vi "EASY-DRIVER Example.vi"() -> ()   [LabVIEW 2020, in "CAENels EASY-DRIVER.lvlib"]
doc: "When the example is executed, it sets the FAST-PS to CV mode and updates the set-point 10 times per second."
uses:
  CAENels EASY-DRIVER.lvlib
panel:
  out "Output Current Chart":dbl(graph)
  out "Fault condition":bool
  out "ON/OFF":bool
  out "Module Status":string="0"
  out "Output Voltage":string="0"
  out "Output Current":string="0"
  in  "Current Setpoint":dbl step=0.1
  in  "Stop Button":bool
  in  "IP address":string="192.168.0.10"
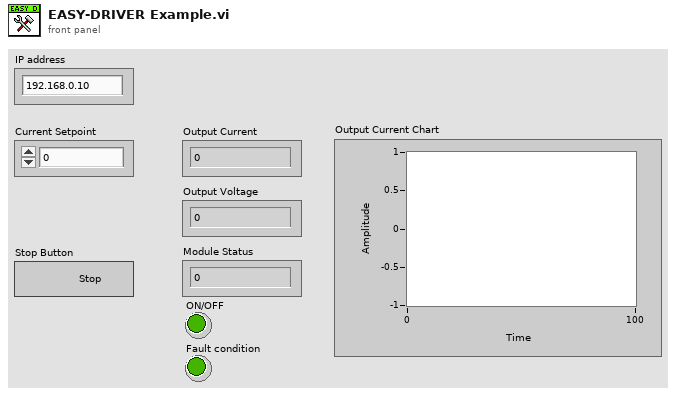
[diagram p1: front panel]
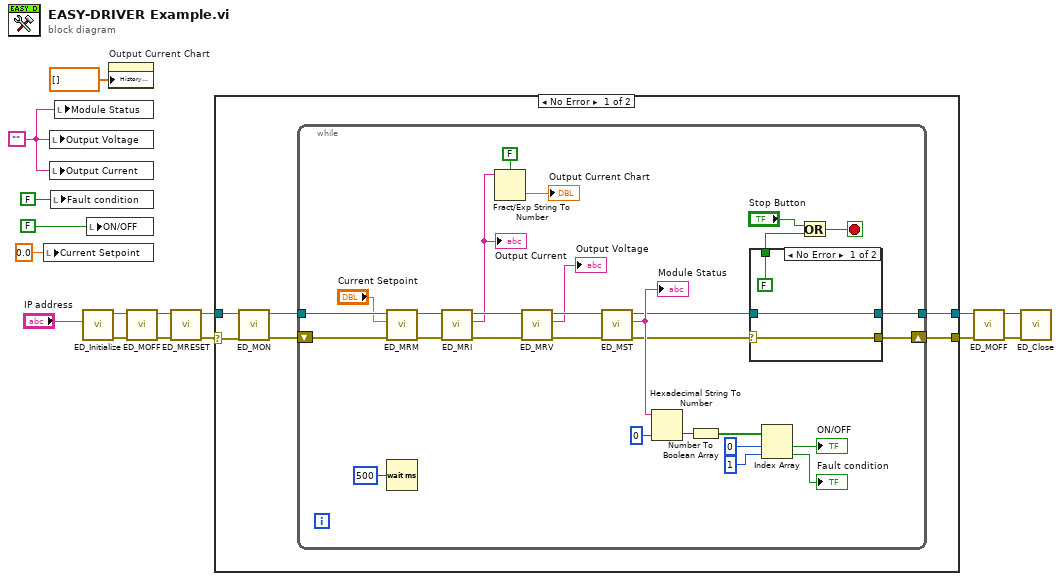
[diagram p0: block diagram]
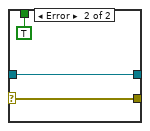
[diagram p2: hidden frame]
diagram:
  w2 = ""
  n1 = local write "Current Setpoint"(0.0 ("Current Setpoint")) -> ()
  n2 = local write "Output Voltage"(w2) -> ()
  n3 = local write "Output Current"(w2) -> ()
  n4 = local write "Fault condition"(FALSE ("Fault condition")) -> ()
  n5 = local write "Module Status"(w2) -> ()
  n6 = call "ED_Initialize.vi"("IP address"="IP address") -> ("error out"=w15:errorcluster, "connection ID"=w14:refnum<k5>)  [unwired: 5 in]
  n7 = local write "ON/OFF"(FALSE ("ON/OFF")) -> ()
  n8 = property on="Output Current Chart" class="WFChart (strict)"("History Data"=dbl[] []) -> ()  [unwired: 2 in, 2 out]
  n9 = call "ED_MOFF.vi"("error in (no error)"=w15, "connection ID"=w14) -> ("error out"=w12:errorcluster, "connection ID out"=w13:refnum<k5>)  [unwired: 4 in]
  n10 = call "ED_MRESET.vi"("error in (no error)"=w12, "connection ID"=w13) -> ("error out"=w3:errorcluster, "connection ID out"=w7:refnum<k5>)  [unwired: 4 in]
  n11 = case shown="No Error" w3 {
    selector: w3 -> [w17 w58]
    tunnel: [w19 w58] -> w9
    tunnel: [w18 w59] -> w8
    tunnel: w7 -> [w22 w59]
    frame No Error {
      n12 = call "ED_MON.vi"("error in (no error)"=w17, "connection ID"=w22) -> ("error out"=w20:errorcluster, "connection ID out"=w21:refnum<k5>)  [unwired: 4 in]
      n13 = while {
        tunnel: w21 -> [w49]
        shift-right: [w31] -> w19
        shift-left: w20 -> [w50]
        tunnel: [w30] -> w18
        stop <- w27 stop-if-true
        n14 = call "ED_MRM.vi"("error in (no error)"=w50, "current"="Current Setpoint", "connection ID"=w49) -> ("error out"=w47:errorcluster, "connection ID out"=w48:refnum<k5>)  [unwired: 3 in]
        n15 = Wait (ms)(milliseconds to wait=u32 500) -> ()  [unwired: 1 out]
        n16 = call "ED_MRI.vi"("error in (no error)"=w47, "connection ID"=w48) -> ("error out"=w45:errorcluster, "current"=w25:string, "connection ID out"=w46:refnum<k5>)  [unwired: 3 in]
        "Output Current" <- w25
        n17 = Fract/Exp String To Number(use system decimal point (T)=FALSE, string=w25) -> (number=→"Output Current Chart":dbl)  [unwired: 2 in, 1 out]
        n18 = call "ED_MRV.vi"("error in (no error)"=w45, "connection ID"=w46) -> ("error out"=w43:errorcluster, "voltage"=→"Output Voltage":string, "connection ID out"=w44:refnum<k5>)  [unwired: 3 in]
        n19 = call "ED_MST.vi"("error in (no error)"=w43, "connection ID"=w44) -> ("error out"=w32:errorcluster, "MST response"=w33:string, "connection ID out"=w29:refnum<k5>)  [unwired: 3 in]
        "Module Status" <- w33
        n20 = Hexadecimal String To Number(string=w33, default (0uL)=u32 0 ("default (0 U32)")) -> (number=w34:u32)  [unwired: 1 in, 1 out]
        n21 = Number To Boolean Array(number=w34) -> (Boolean array=w39:bool[])
        n22 = case shown="No Error" w32 {
          selector: w32 -> [w54 w55]
          tunnel: [w54 w55] -> w31
          tunnel: [w53 w56] -> w30
          tunnel: w29 -> [w53 w56]
          tunnel: [FALSE TRUE] -> w26
          frame No Error {
          }
          frame Error {
          }
        }
        n23 = Index Array(array=w39, index #1=0 ("index"), index #2=1 ("index")) -> (element #1=→"ON/OFF":bool, element #2=→"Fault condition":bool)
        n24 = Or(x="Stop Button", y=w26) -> (x .or. y?=w27:bool)
      }
    }
    frame Error {
    }
  }
  n25 = call "ED_MOFF.vi"("error in (no error)"=w9, "connection ID"=w8) -> ("error out"=w10:errorcluster, "connection ID out"=w11:refnum<k5>)  [unwired: 4 in]
  n26 = call "ED_Close.vi"("error in (no error)"=w10, "connection ID"=w11) -> ()  [unwired: 5 in, 1 out]
